vi "User Event Driver.vi"(11 "error in":errorcluster, 13 "LV2 Operation":T1) -> (4 "User Event Reference":refnum<user-event>, 15 "error out":errorcluster)   [LabVIEW 2021, in "Game of Life.lvlib" / "User Event.lvlib"]
uses:
  User Event.lvlib
  controls/User Event Operations.ctl
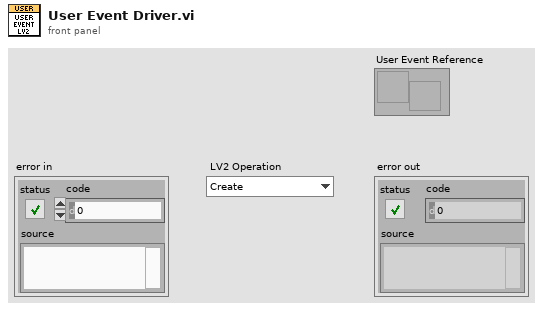
[diagram p1: front panel]
types:
  T1 = typedef "Game of Life.lvlib/User Event.lvlib/User Event Operations.ctl" = enum16{"Create", "Destroy", "Get Reference", "Generate"}
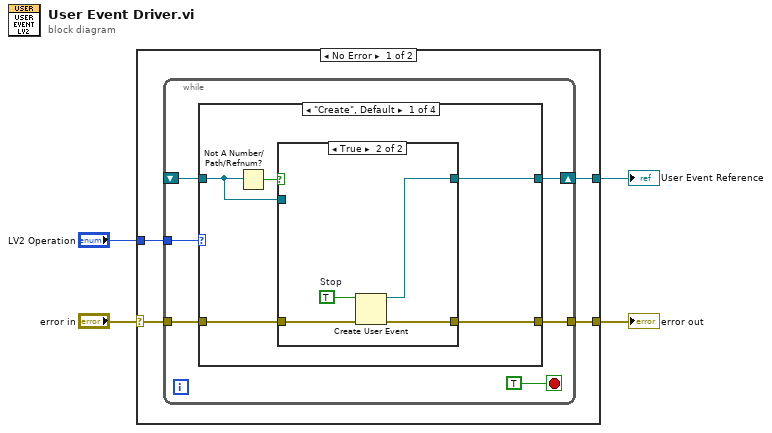
[diagram p0: block diagram]
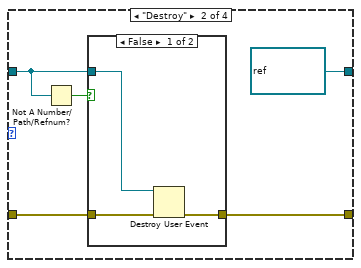
[diagram p3: hidden frame]
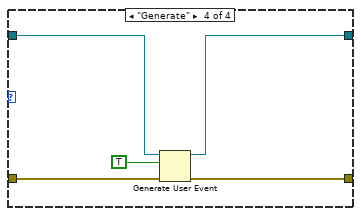
[diagram p6: hidden frame]
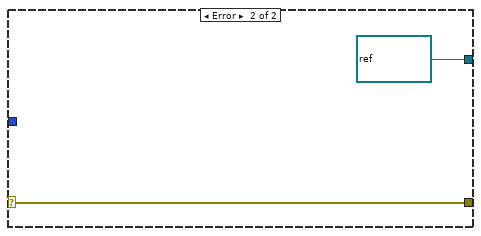
[diagram p7: hidden frame]
diagram:
  n1 = case shown="No Error" "error in" {
    selector: "error in" -> [w8 w43]
    tunnel: [w7 w43] -> w3
    tunnel: "LV2 Operation" -> [w6 _]
    tunnel: [w5 refnum<user-event> refnum ("Data")] -> w1
    frame No Error {
      n2 = while {
        tunnel: w8 -> [w14]
        tunnel: [w13] -> w7
        tunnel: w6 -> [w11]
        shift-right: [w10] -> w5
        shift-left: _ -> [w9]
        stop <- TRUE stop-if-true
        n3 = case shown="\"Create\", Default" w11 {
          tunnel: [w18 w29 w35 w40] -> w13
          tunnel: w14 -> [w19 w30 w35 w41]
          tunnel: [w17 refnum<user-event> refnum ("Data") w36 w38] -> w10
          tunnel: w9 -> [w15 w27 w36 w39]
          frame "Create", Default {
            n4 = Not A Number/Path/Refnum?(number/path/refnum=w15) -> (NaN/Path/Refnum?=w16:bool)
            n5 = case shown="True" w16 {
              tunnel: w19 -> [w20 w25]
              tunnel: [w20 w24] -> w18
              tunnel: [w21 w23] -> w17
              tunnel: w15 -> [w21 _]
              frame False {
              }
              frame True {
                w22 = TRUE  # Stop
                n6 = Create User Event(user event datatype=w22, error in=w25) -> (user event=w23:refnum<user-event>, error out=w24:errorcluster)
              }
            }
          }
          frame "Destroy" {
            n7 = Not A Number/Path/Refnum?(number/path/refnum=w27) -> (NaN/Path/Refnum?=w28:bool)
            n8 = case shown="False" w28 {
              tunnel: w30 -> [w32 w34]
              tunnel: [w31 w34] -> w29
              tunnel: w27 -> [w33 _]
              frame False {
                n9 = Destroy User Event(user event=w33, error in=w32) -> (error out=w31:errorcluster)
              }
              frame True {
              }
            }
          }
          frame "Get Reference" {
          }
          frame "Generate" {
            n10 = Generate User Event(user event=w39, event data cluster=TRUE ("event data"), error in=w41) -> (user event out=w38:refnum<user-event>, error out=w40:errorcluster)  [unwired: 1 in]
          }
        }
      }
    }
    frame Error {
    }
  }
  "error out" <- w3
  "User Event Reference" <- w1
